vi "RSZVB Get Dummy Source Power Calibration State.vi"(8 "error in (no error)":errorcluster {"code" format="%.0x"}, 9 "Port Number (1)":i32=1, 10 "Channel (1)":i32=1, 11 "VISA session":refnum<visa-resource-name>) -> (0 "error out":errorcluster {"code" format="%.0x"}, 1 "Dummy Source Power Calibration":bool, 3 "dup VISA session":refnum<visa-resource-name>)   [LabVIEW 2011]
doc: "This VI returns whether dummy or real source power calibration is selected\n\nRemote-control command(s):\nSOURce<Ch>:POWer<Pt>:CORRection:DEFault?"
uses:
  _utility/RSZVB Global Data.vi
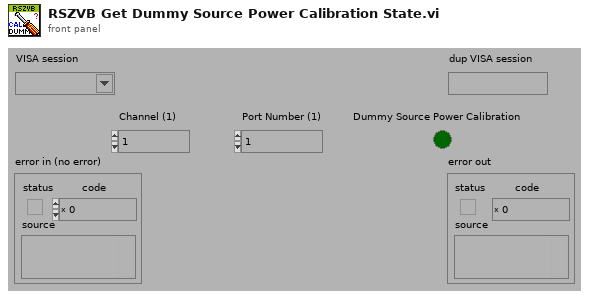
[diagram p1: front panel]
types:
  T1 = cluster{"Error Checking (T: On)":bool, "Installed Options":string[], "Data Valid?":bool, "Ports":i32, "Model":string[], "Option Checking (T: On)":bool}[]
  T2 = cluster{"Error Checking (T: On)":bool, "Installed Options":string[], "Data Valid?":bool, "Ports":i32, "Model":string[], "Option Checking (T: On)":bool}
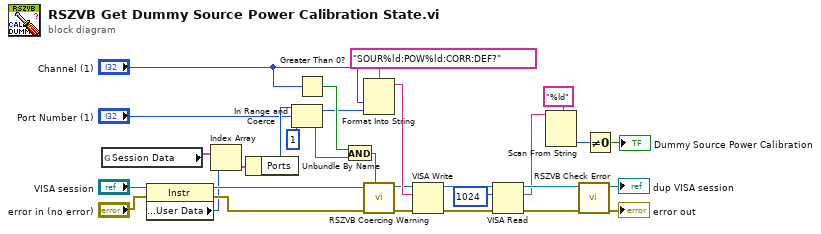
[diagram p0: block diagram]
diagram:
  n1 = global read "RSZVB Global Data.vi" "Session Data"() -> (w19:T1)
  n2 = property class="Instr"(reference="VISA session", error in="error in (no error)") -> (reference out=w21:refnum<visa-resource-name>, error out=w30:errorcluster, "General Settings:User Data"=w18:u32)
  n3 = Index Array(array=w19, index=w18) -> (element=w20:T2)
  n4 = Unbundle By Name(w20) -> ("Ports"=w22:i32)
  n5 = In Range and Coerce(upper limit=w22, x="Port Number (1)", lower limit=1) -> (coerced(x)=w24:i32, In Range?=w27:bool)
  n6 = Greater Than 0?(x="Channel (1)") -> (x > 0?=w28:bool)
  n7 = And(x=w28, y=w27) -> (x .and. y?=w25:bool)
  n8 = Format Into String(format string="SOUR%ld:POW%ld:CORR:DEF?", "Channel (1)", w24) -> (resulting string=w29:string)  [unwired: 2 in, 1 out]
  n9 = call "RSZVB Coercing Warning.vi"("In Range?"=w25, "error in (no error)"=w30, "VISA session"=w21) -> ("error out"=w16:errorcluster, "dup VISA session"=w26:refnum<visa-resource-name>)  [unwired: 7 in]
  n10 = VISA Write(VISA resource name=w26, write buffer=w29, error in (no error)=w16) -> (VISA resource name out=w10:refnum<visa-resource-name>, error out=w9:errorcluster)  [unwired: 1 out]
  n11 = VISA Read(VISA resource name=w10, byte count=u32 1024 ("byte count (0)"), error in (no error)=w9) -> (VISA resource name out=w6:refnum<visa-resource-name>, read buffer=w1:string, error out=w12:errorcluster)  [unwired: 1 out]
  n12 = Scan From String(format string="%ld", input string=w1) -> (output 1=w3:i32)  [unwired: 3 in, 3 out]
  n13 = call "RSZVB Check Error.vi"("error in (no error)"=w12, "VISA session"=w6) -> ("error out"=→"error out":errorcluster, "dup VISA session"=→"dup VISA session":refnum<visa-resource-name>)  [unwired: 8 in]
  n14 = Not Equal To 0?(x=w3) -> (x != 0?=→"Dummy Source Power Calibration":bool)
